vi "FTW-JSON-Object-Join.vi"(0 "JSON Object":refnum<data-value>, 5 "JSON Object to Merge":refnum<data-value>, 7 "Join Mode":T1, 11 "error in":errorcluster) -> (4 "JSON Object out":refnum<data-value>, 15 "error out":errorcluster)   [LabVIEW 2015]
uses:
  core/FTW-JSON-Core-Structure.ctl
  FTW-JSON-UpdateMode.ctl
panel:
  # "Inputs"
  # "Outputs"
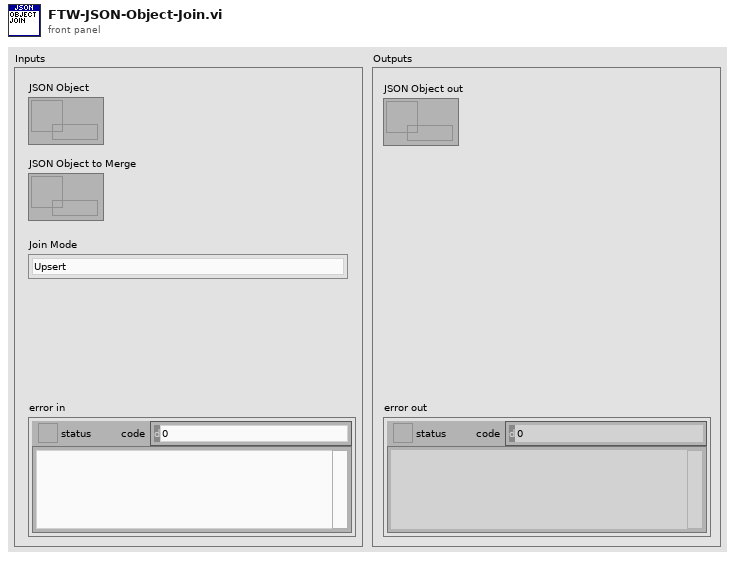
[diagram p1: front panel]
types:
  T1 = typedef "FTW-JSON-UpdateMode.ctl" = enum32{"Upsert", "Update Only", "Insert Only"}
  T2 = typedef "FTW-JSON-Core-Structure.ctl" = cluster{"JSON Object":i64, "Encoding Flags":i64, "Decoding Flags":i64}
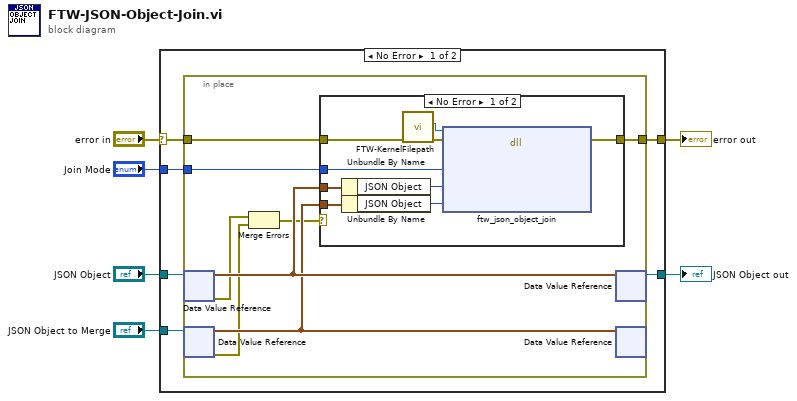
[diagram p0: block diagram]
diagram:
  n1 = case shown="No Error" "error in" {
    selector: "error in" -> [w12 w32]
    tunnel: [w11 w32] -> w6
    tunnel: [w8 w31] -> w4
    tunnel: "JSON Object" -> [w9 w31]
    tunnel: "JSON Object to Merge" -> [w7 _]
    tunnel: "Join Mode" -> [w10 _]
    frame No Error {
      n2 = in-place {
        in-place-border: w12 -> [w18]
        in-place-border: [w19] -> w11
        in-place-border: w10 -> [w20]
        n3 = in-place-dvr #1(w9) -> (w17:T2, w14:errorcluster)
        n4 = in-place-dvr #2(w7) -> (w16:T2, w13:errorcluster)
        n5 = Merge Errors(w14, w13) -> (w15:errorcluster)
        n6 = case shown="No Error" w15 {
          tunnel: w20 -> [w24 _]
          tunnel: [w28 w30] -> w19
          tunnel: w18 -> [w23 w30]
          tunnel: w17 -> [w26 _]
          tunnel: w16 -> [w25 _]
          frame No Error {
            n7 = Unbundle By Name(w26) -> ("JSON Object"=w27:i64)
            n8 = Unbundle By Name(w25) -> ("JSON Object"=w29:i64)
            n9 = call "FTW-KernelFilepath.vi"("error in"=w23) -> ("error out"=w22:errorcluster, "Library Filepath"=w21:path)  [unwired: 8 in, 1 out]
            n10 = dll-call lib="?" fn="ftw_json_object_join"(path in=w21, error in=w22, "Join Mode"=w24, "JSON Object ID"=w27, "JSON Object ID to Merge"=w29) -> (error out=w28:errorcluster)  [unwired: 5 in, 1 out]
          }
          frame Error {
          }
        }
        n11 = in-place-dvr #1(w17) -> (w8:refnum<data-value>)  [unwired: 1 out]
        n12 = in-place-dvr #2(w16) -> ()  [unwired: 2 out]
      }
    }
    frame Error {
    }
  }
  "error out" <- w6
  "JSON Object out" <- w4
